vi "例9.2 采集一段声音快速VI.vi"() -> ()   [LabVIEW 2017]
panel:
  in  "Duration (s)":dbl=1.0 caption="持续时间(s)"
  out "采集的波形":dynamicdata(graph)
  in  "Resolution (bits)":i32=16 caption="分辨率（位）"
  in  "#Channels":i32=2 caption="通道数量"
  in  "Sample rate (Hz)":dbl=44100.0 caption="采样率(Hz)"
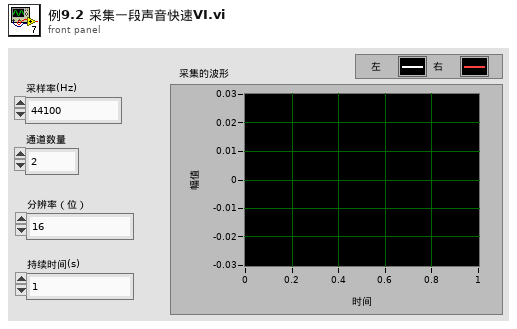
[diagram p1: front panel]
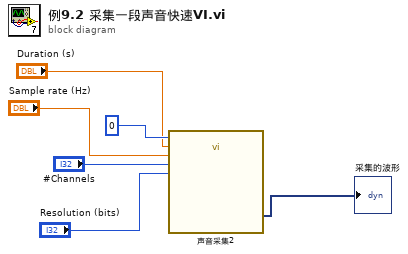
[diagram p0: block diagram]
diagram:
  n1 = call "声音采集2"("Device"=u32 0, "Duration (s)"="Duration (s)", "Sample rate (Hz)"="Sample rate (Hz)", "#Channels"="#Channels", "Resolution (bits)"="Resolution (bits)") -> ("Data"=→"采集的波形":dynamicdata)  [unwired: 13 in, 1 out]
